vi "UserDefined.Compile.vi"(8 "error in (no error)":errorcluster, 11 "Section Ref in":T4 format="%.0x") -> (0 "error out":errorcluster, 2 "Settings":T1 {"Signal.Cmd.Refs"."Signal Refs" format="%.0x"; "Signal.Cmd.Info"."Signals"."Byte Order" items=["Little Endian", "Big Endian"]; "Signal.Cmd.Info"."Signals"."Data Type" items=["Signed", "Unsigned", "IEEE Float"]; "Settings.Refs"."Signal Refs" format="%.0x"; "Signal.Resp.Refs"."Signal Refs" format="%.0x"; "Signal.Resp.Info"."Signals"."Byte Order" items=["Little Endian", "Big Endian"]; "Signal.Resp.Info"."Signals"."Data Type" items=["Signed", "Unsigned", "IEEE Float"]; "Trigger.Refs"."Signal Refs" format="%.0x"; "Status.Refs"."Signal Refs" format="%.0x"}, 3 "Section Ref out":T4 format="%.0x")   [LabVIEW 2019, in "Diagnostics Addon System Explorer.lvlib"]
uses:
  Diagnostics Addon System Explorer.lvlib
  <vilib>/NI VeriStand/Custom Device Tools/Custom Device Utility Library/Custom Device Utility Library.lvlib
  <vilib>/NI VeriStand/Custom Device Tools/Custom Device Utility Library/NI VeriStand - Search for Item by GUID.vi
  <vilib>/NI VeriStand/Custom Device API/Custom Device Item Ref.ctl
  <vilib>/NI VeriStand/Custom Device API/Custom Device API.lvlib
  Shared/Types/Signal.ctl
  Shared/Diagnostics Addon Shared.lvlib
  Shared/Types/Frame.Compile.ctl
  Shared/SubVIs/Constants.vi
  Types/FG.Action.ctl
  Types/Frame.Ref.ctl
  Shared/Types/Type.ctl
  <vilib>/NI VeriStand/Custom Device Tools/Custom Device Utility Library/NI VeriStand - Search for All Items by GUID.vi
  Types/Service.Export.ctl
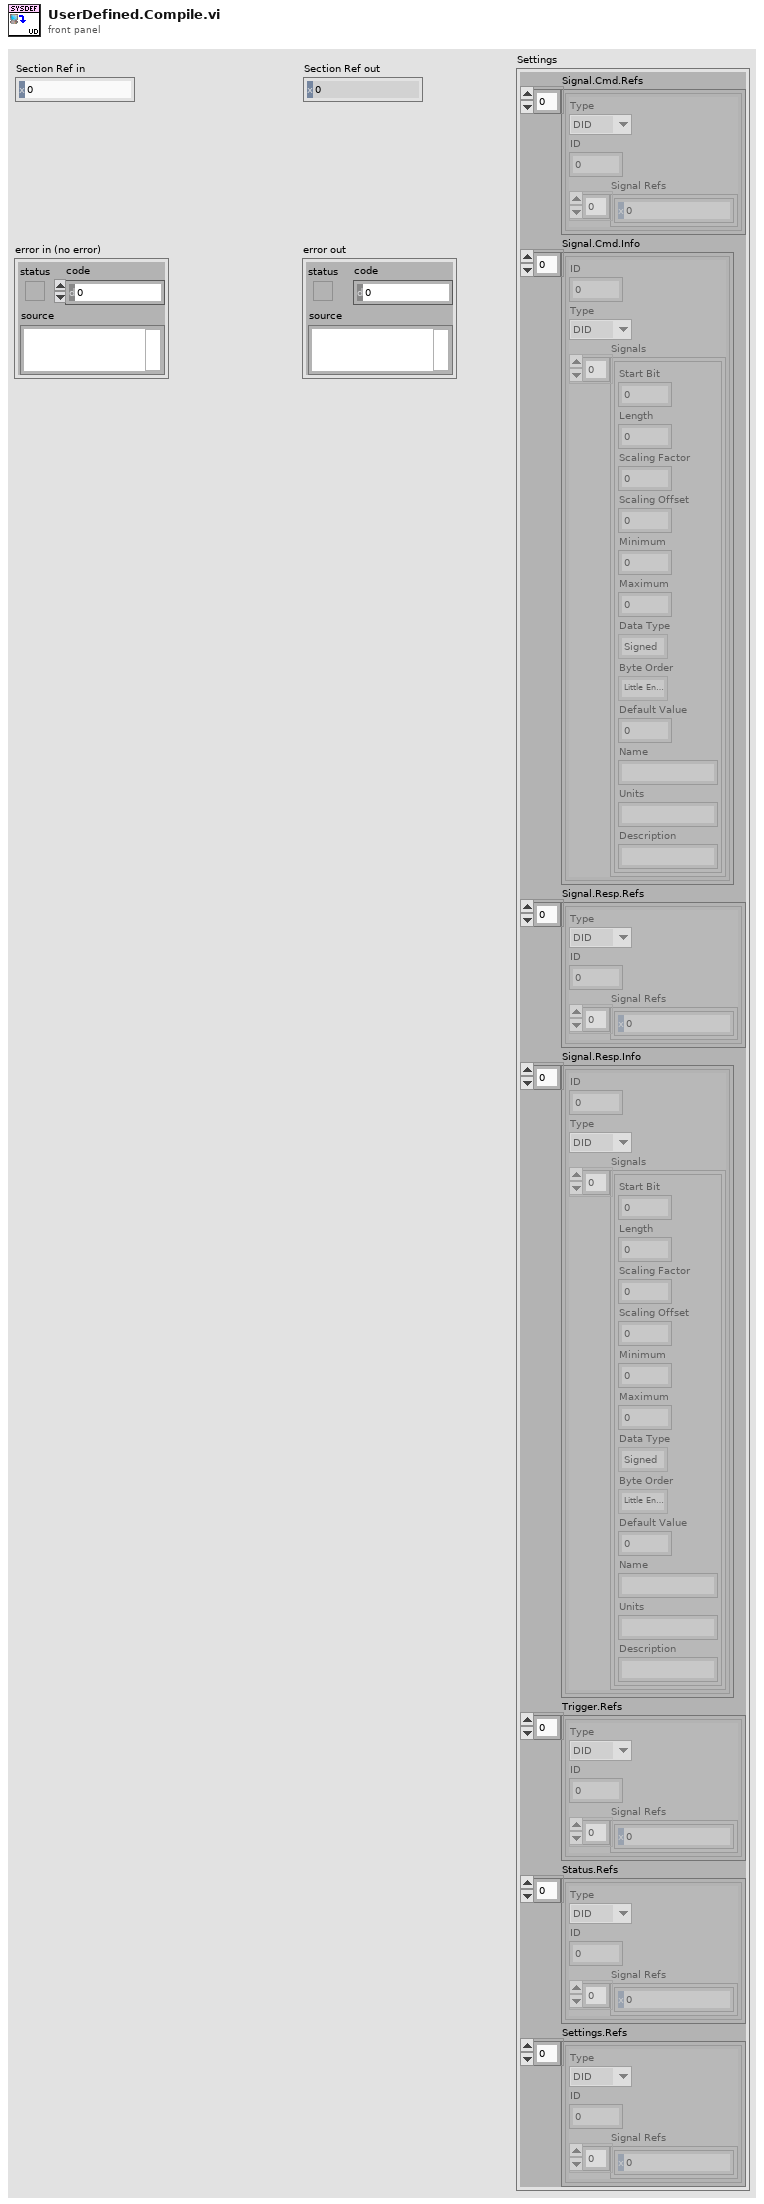
[diagram p1: front panel]
types:
  T1 = typedef "Diagnostics Addon System Explorer.lvlib/Service.Export.ctl" = cluster{"Signal.Cmd.Refs":T2[], "Signal.Cmd.Info":T5[], "Signal.Resp.Refs":T2[], "Signal.Resp.Info":T5[], "Trigger.Refs":T2[], "Status.Refs":T2[], "Settings.Refs":T2[]}
  T2 = typedef "Diagnostics Addon System Explorer.lvlib/Frame.Ref.ctl" = cluster{"Type":T3, "ID":u32, "Signal Refs":T4[]}
  T3 = typedef "Diagnostics Addon Shared.lvlib/Type.ctl" = enum16{"DID", "CDID", "PID", "CPID", "Read Memory", "Write Memory", "DTC Control", "IO Cmd", "IO Resp", "Routine Start Cmd", "Routine Start Resp", "Routine Request Cmd", "Routine Request Resp", "Routine Stop Cmd", "Routine Stop Resp", "UserDefined Cmd", "UserDefined Rsp", "Tester Present", "Clear DTCs", "Read DTCs", "Start DTCs", "DTC Change Count", "Unlock ECU", "Reset ECU", "Diagnostic Session Control", "Normal Communication Control", "Configure and Start DPIDs", "Stop DPIDs"}
  T4 = typedef "Custom Device API.lvlib/Custom Device Item Ref.ctl" = u64
  T5 = typedef "Diagnostics Addon Shared.lvlib/Frame.Compile.ctl" = cluster{"ID":u32, "Type":T3, "Signals":T6[]}
  T6 = typedef "Diagnostics Addon Shared.lvlib/Signal.ctl" = cluster{"Start Bit":u32, "Length":u32, "Scaling Factor":dbl, "Scaling Offset":dbl, "Minimum":dbl, "Maximum":dbl, "Data Type":u32, "Byte Order":u32, "Default Value":dbl, "Name":string, "Units":string, "Description":string}
  T7 = typedef "Diagnostics Addon System Explorer.lvlib/FG.Action.ctl" = enum16{"Get", "Set"}
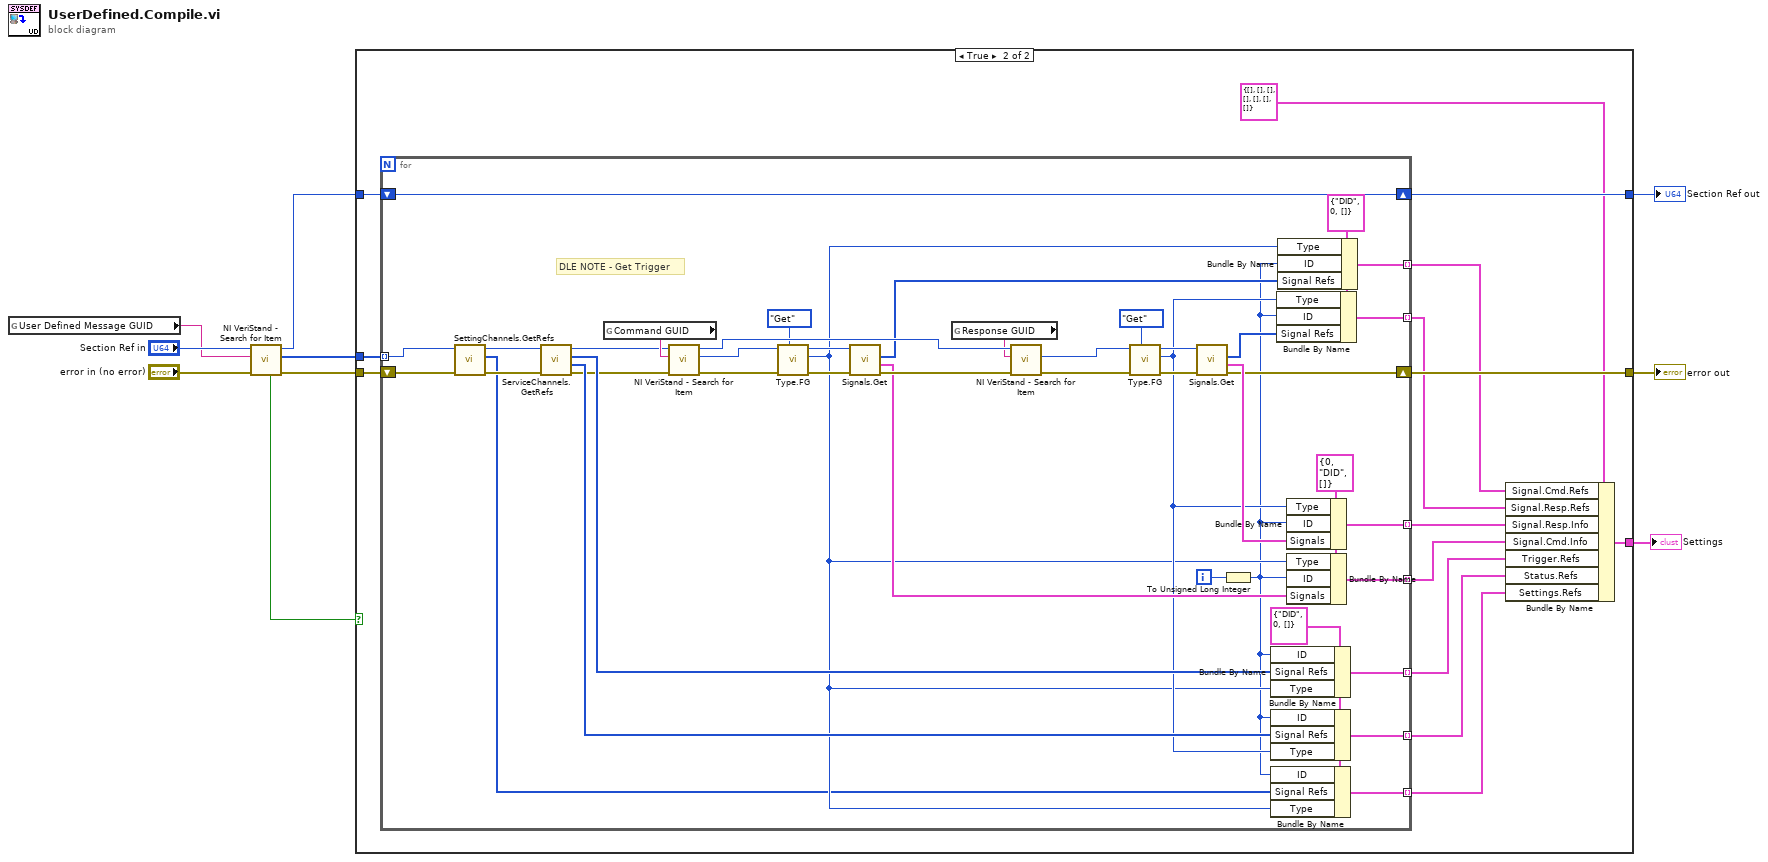
[diagram p0: block diagram]
diagram:
  n1 = global read "Constants.vi" "User Defined Message GUID"() -> (w4:string)
  n2 = call-poly <vilib>:"NI VeriStand - Search for Item.vi"("error in"="error in (no error)", "Item GUID"=w4, "Section Ref in"="Section Ref in") -> ("error out"=w6:errorcluster, "Item Refs"=w7:T4[], "Section Ref out"=w3:T4, "Found"=w5:bool)  [unwired: 5 in]
  n3 = case shown="True" w5 {
    tunnel: [w12 w26] -> w10
    tunnel: w7 -> [_ w24]
    tunnel: w6 -> [w12 w25]
    tunnel: w3 -> [w11 w23]
    tunnel: [w11 w22] -> w2
    tunnel: [_ w14] -> w1
    frame False {
    }
    frame True {
      n4 = for {
        shift-right: [w62] -> w26
        shift-left: w25 -> [w35]
        tunnel: w24 -> [w32] mode=indexing
        tunnel: [w61] -> w18 mode=indexing
        tunnel: [w60] -> w17 mode=indexing
        tunnel: [w56] -> w20 mode=indexing
        tunnel: [w55] -> w19 mode=indexing
        shift-right: [w44] -> w22
        shift-left: w23 -> [w44]
        tunnel: [w40] -> w16 mode=indexing
        tunnel: [w39] -> w15 mode=indexing
        tunnel: [w31] -> w13 mode=indexing
        i -> [w41]
        w30 = T2 {"Type"=enum."DID", "ID"=0, "Signal Refs"=[]} ("cluster")
        w58 = T2 {"Type"=enum."DID", "ID"=0, "Signal Refs"=[]} ("Cmd")
        w69 = T5 {"ID"=0, "Type"=enum."DID", "Signals"=[]} ("PID In")
        # "DLE NOTE - Get Trigger"
        n5 = call "SettingChannels.GetRefs.vi"("error in (no error)"=w35, "Item Ref in"=w32) -> ("error out"=w34:errorcluster, "Settings"=w27:T4[], "Section Ref out"=w33:T4)  [unwired: 7 in]
        n6 = call "ServiceChannels.GetRefs.vi"("error in (no error)"=w34, "Item Ref in"=w33) -> ("error out"=w36:errorcluster, "Status"=w43:T4[], "Trigger"=w42:T4[], "Section Ref out"=w37:T4)  [unwired: 6 in]
        n7 = global read "Constants.vi" "Command GUID"() -> (w65:string)
        n8 = call-poly <vilib>:"NI VeriStand - Search for Item.vi"("error in"=w36, "Item GUID"=w65, "Section Ref in"=w37) -> ("error out"=w54:errorcluster, "Item Ref"=w52:T4, "Section Ref out"=w67:T4)  [unwired: 5 in, 1 out]
        n9 = call "Type.FG.vi"("Action"=FG.Action."Get", "error in (no error)"=w54, "Device Item Ref in"=w52) -> ("error out"=w53:errorcluster, "Type"=w29:T3, "Device Item Ref out"=w51:T4)  [unwired: 6 in]
        n10 = call "Signals.Get.vi"("error in (no error)"=w53, "Device Item Ref out"=w51) -> ("error out"=w68:errorcluster, "Parameters"=w64:T6[], "Child Refs"=w59:T4[])  [unwired: 6 in, 1 out]
        n11 = global read "Constants.vi" "Response GUID"() -> (w66:string)
        n12 = call-poly <vilib>:"NI VeriStand - Search for Item.vi"("error in"=w68, "Item GUID"=w66, "Section Ref in"=w67) -> ("error out"=w48:errorcluster, "Item Ref"=w46:T4)  [unwired: 5 in, 2 out]
        n13 = call "Type.FG.vi"("Action"=FG.Action."Get", "error in (no error)"=w48, "Device Item Ref in"=w46) -> ("error out"=w47:errorcluster, "Type"=w38:T3, "Device Item Ref out"=w45:T4)  [unwired: 6 in]
        n14 = call "Signals.Get.vi"("error in (no error)"=w47, "Device Item Ref out"=w45) -> ("error out"=w62:errorcluster, "Parameters"=w63:T6[], "Child Refs"=w57:T4[])  [unwired: 6 in, 1 out]
        n15 = To Unsigned Long Integer(number=w41) -> (unsigned 32bit integer=w28:u32)
        n16 = Bundle By Name(cluster=w30, "ID"=w28, "Signal Refs"=w42, "Type"=w29) -> (w40:T2)
        n17 = Bundle By Name(cluster=w30, "ID"=w28, "Signal Refs"=w43, "Type"=w38) -> (w39:T2)
        n18 = Bundle By Name(cluster=w30, "ID"=w28, "Signal Refs"=w27, "Type"=w29) -> (w31:T2)
        n19 = Bundle By Name(cluster=w58, "Type"=w38, "ID"=w28, "Signal Refs"=w57) -> (w55:T2)
        n20 = Bundle By Name(cluster=w58, "Type"=w29, "ID"=w28, "Signal Refs"=w59) -> (w56:T2)
        n21 = Bundle By Name(cluster=w69, "Type"=w38, "ID"=w28, "Signals"=w63) -> (w61:T5)
        n22 = Bundle By Name(cluster=w69, "Type"=w29, "ID"=w28, "Signals"=w64) -> (w60:T5)
      }
      n23 = Bundle By Name(cluster=T1 {"Signal.Cmd.Refs"=[], "Signal.Cmd.Info"=[], "Signal.Resp.Refs"=[], "Signal.Resp.Info"=[], "Trigger.Refs"=[], "Status.Refs"=[], "Settings.Refs"=[]} ("Settings"), "Signal.Cmd.Refs"=w20, "Signal.Resp.Refs"=w19, "Signal.Resp.Info"=w18, "Signal.Cmd.Info"=w17, "Trigger.Refs"=w16, "Status.Refs"=w15, "Settings.Refs"=w13) -> (w14:T1)
    }
  }
  "Section Ref out" <- w2
  "error out" <- w10
  "Settings" <- w1
